vi "Pick A DOF.vi"(6 "LBCB Number":T1, 7 "Force Control Parameters":T3, 8 "error in (no error)":errorcluster, 9 "Force Group Priorities":T4, 10 "Forces Error \nWindow":dbl[](array[numeric]), 11 "Mixed Mode Convergence Status In":T2) -> (0 "error out":errorcluster, 3 "Mixed Mode Convergence Status Out":T2)   [LabVIEW 2009]
uses:
  Data Access Objects/Metadata/Cartesian Point.ctl
  Data Access Objects/Mixed Mode/Force Control Parameters.ctl
  Mixed Mode Convergence Status.ctl
  Data Access Objects/Metadata/LBCB Number.ctl
  Data Access Objects/Metadata/DAO Actions.ctl
  Apps/Yes No Button.ctl
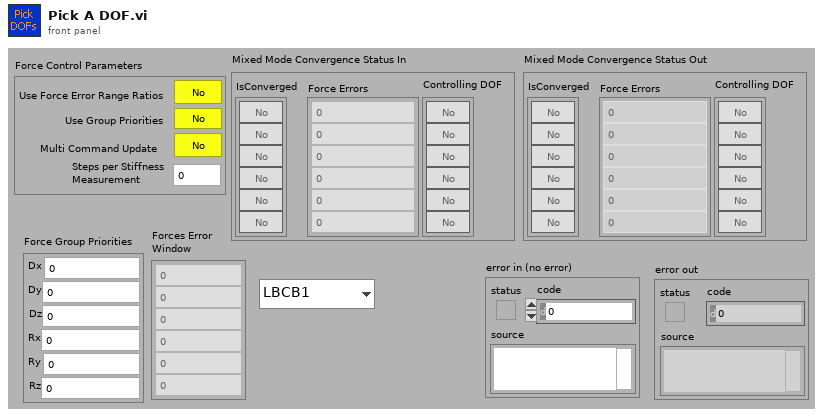
[diagram p1: front panel]
types:
  T1 = typedef "LBCB Number.ctl" = enum16{"LBCB1", "LBCB2"}
  T2 = typedef "Mixed Mode Convergence Status.ctl" = cluster{"IsConverged":bool[], "Force Errors":dbl[], "Controlling DOF":bool[]}
  T3 = typedef "Force Control Parameters.ctl" = cluster{"Use Force Error Range Ratios":bool, "Use Group Priorities":bool, "Multi Command Update":bool, "Steps per Stiffness \nMeasurement":i32}
  T4 = typedef "Cartesian Point.ctl" = cluster{"Dx":dbl, "Dy":dbl, "Dz":dbl, "Rx":dbl, "Ry":dbl, "Rz":dbl}
  T5 = typedef "Pick A DOF Strategy Types.ctl" = enum16{"Absolute Force Error", "Normalized Force Error", "Group Priorities Absolute", "Group Priorities Normalized", "Multi DOF Ramp Counting", "Multi DOF Ramp Counting Group", "Multi DOF Stiffness Test"}
  T6 = typedef "DAO Actions.ctl" = enum16{"Init", "Get", "Set"}
  T7 = typedef "Yes No Button.ctl" = bool
  T8 = typedef "Mixed Mode Multidof Status.ctl" = cluster{"Mixed Mode Multidof State":T9, "Multi DOF Ramp Count":i32, "Stiffness Tested":T7[][]}
  T9 = typedef "Mixed Mode Multidof State.ctl" = enum16{"Multidof", "Stiffness Test"}
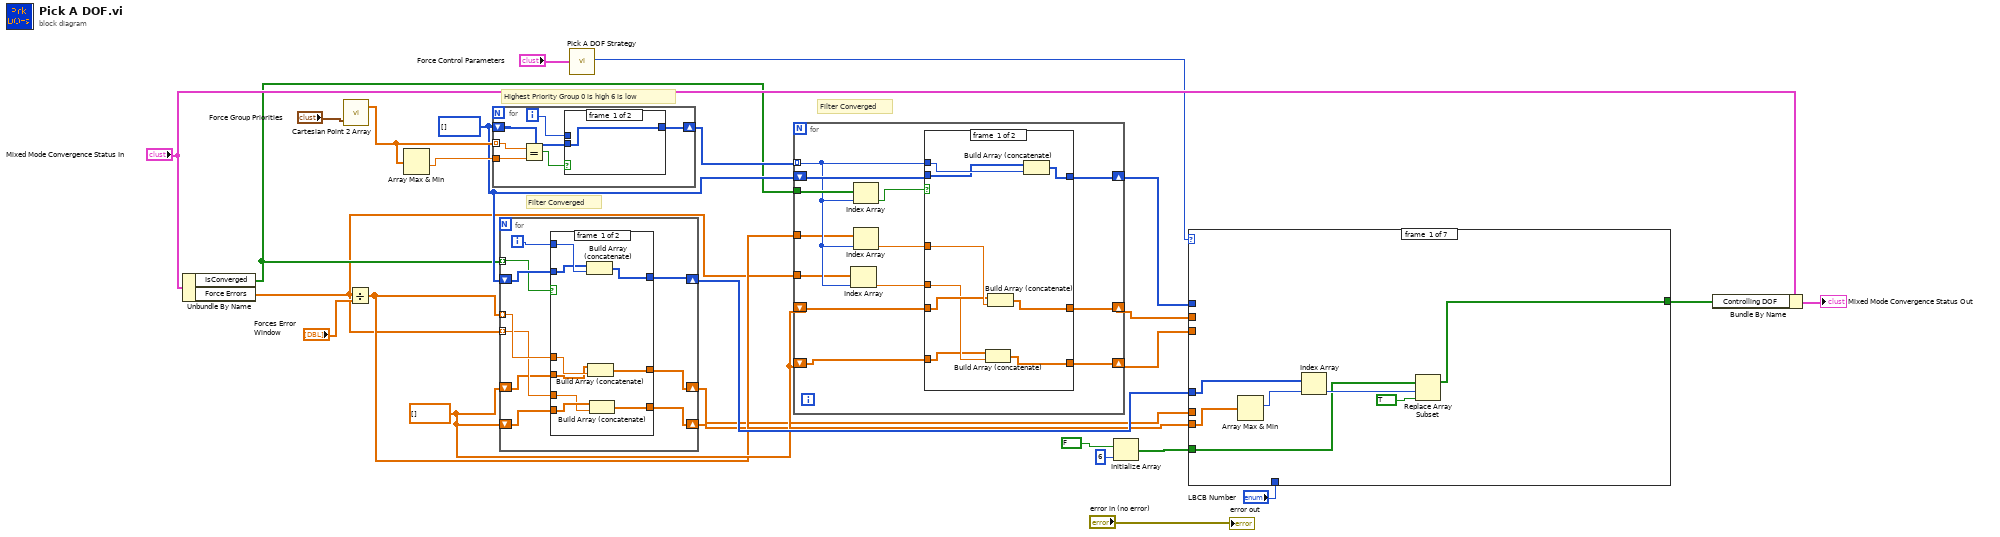
[diagram p0: block diagram]
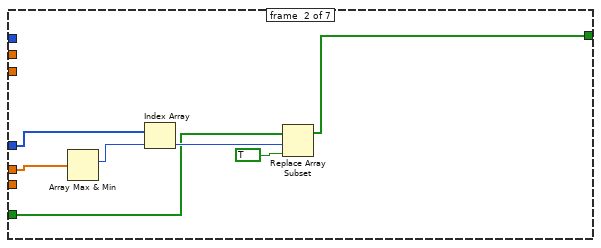
[diagram p2: hidden frame]
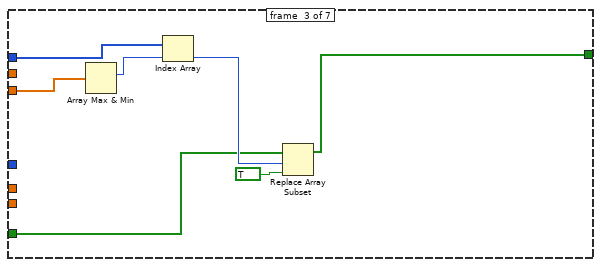
[diagram p3: hidden frame]
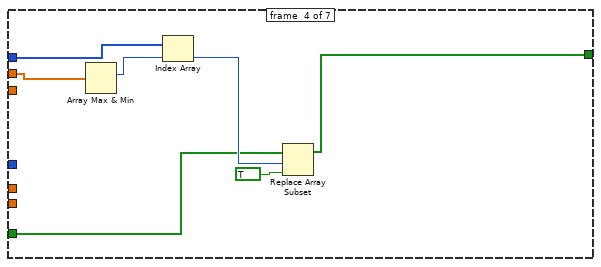
[diagram p4: hidden frame]
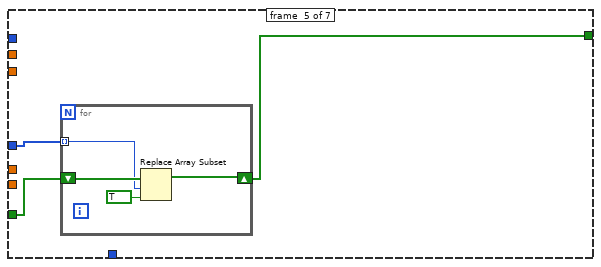
[diagram p5: hidden frame]
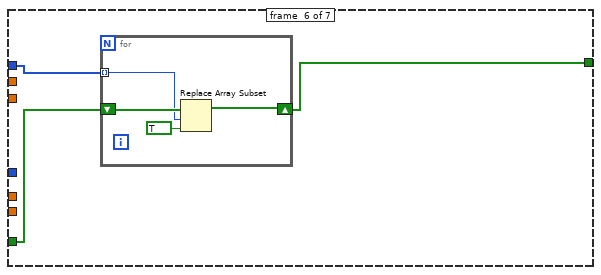
[diagram p6: hidden frame]
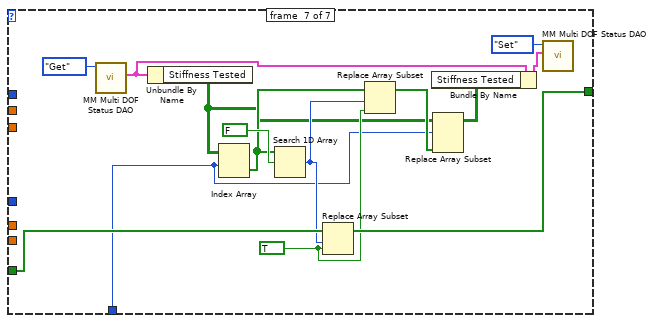
[diagram p7: hidden frame]
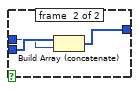
[diagram p10: hidden frame]
diagram:
  w10 = dbl[] []
  w17 = i32[] []
  # "Filter Converged"
  # "Filter Converged"
  # "Highest Priority Group 0 is high 6 is low"
  n1 = Unbundle By Name("Mixed Mode Convergence Status In") -> ("IsConverged"=w16:bool[], "Force Errors"=w1:dbl[])
  n2 = call "Cartesian Point 2 Array.vi"("Cart Disp"="Force Group Priorities") -> ("Array"=w20:dbl[])  [unwired: 2 in]
  n3 = Divide(x=w1, y="Forces Error \nWindow") -> (x/y=w9:dbl[])
  n4 = Array Max & Min(array=w20) -> (min value=w19:dbl)  [unwired: 3 out]
  n5 = for {
    shift-right: [w27] -> w18
    shift-left: w17 -> [w29]
    tunnel: w20 -> [w31] mode=indexing
    tunnel: w19 -> [w32]
    i -> [w28]
    n6 = Equal?(x=w31, y=w32) -> (x = y?=w30:bool)
    n7 = case shown="True" w30 {
      tunnel: w29 -> [w33 w35]
      tunnel: w28 -> [_ w34]
      tunnel: [w33 w36] -> w27
      frame #0 {
      }
      frame #1 {
        n8 = Build Array (concatenate)(w35, w34) -> (w36:i32[])
      }
    }
  }
  n9 = for {
    shift-right: [w44] -> w11
    shift-left: w17 -> [w45]
    tunnel: w16 -> [w43] mode=indexing
    shift-right: [w37] -> w5
    shift-left: w10 -> [w40]
    shift-right: [w38] -> w4
    shift-left: w10 -> [w39]
    tunnel: w9 -> [w42] mode=indexing
    tunnel: w1 -> [w41] mode=indexing
    i -> [w46]
    n10 = case shown="False" w43 {
      tunnel: w45 -> [w51 w58]
      tunnel: w46 -> [w52 _]
      tunnel: [w55 w58] -> w44
      tunnel: w42 -> [w50 _]
      tunnel: w41 -> [w47 _]
      tunnel: w40 -> [w49 w57]
      tunnel: w39 -> [w48 w56]
      tunnel: [w54 w56] -> w38
      tunnel: [w53 w57] -> w37
      frame #0 {
        n11 = Build Array (concatenate)(w51, w52) -> (w55:i32[])
        n12 = Build Array (concatenate)(w49, w50) -> (w53:dbl[])
        n13 = Build Array (concatenate)(w48, w47) -> (w54:dbl[])
      }
      frame #1 {
      }
    }
  }
  n14 = call "Pick A DOF Strategy.vi"("Force Control Parameters"="Force Control Parameters") -> ("Pick A DOF Strategy"=w14:T5)  [unwired: 10 in]
  n15 = for {
    tunnel: w16 -> [w69]
    tunnel: w18 -> [w67] mode=indexing
    shift-right: [w70] -> w12
    shift-left: w17 -> [w71]
    shift-right: [w59] -> w7
    shift-left: w10 -> [w62]
    shift-right: [w60] -> w6
    shift-left: w10 -> [w61]
    tunnel: w9 -> [w66]
    tunnel: w1 -> [w65]
    n16 = Index Array(array=w65, index=w67) -> (element=w63:dbl)
    n17 = Index Array(array=w69, index=w67) -> (element=w68:bool)
    n18 = Index Array(array=w66, index=w67) -> (element=w64:dbl)
    n19 = case shown="False" w68 {
      tunnel: w71 -> [w76 w83]
      tunnel: w67 -> [w77 _]
      tunnel: [w80 w83] -> w70
      tunnel: w64 -> [w75 _]
      tunnel: w63 -> [w73 _]
      tunnel: w62 -> [w74 w82]
      tunnel: w61 -> [w72 w81]
      tunnel: [w79 w81] -> w60
      tunnel: [w78 w82] -> w59
      frame #0 {
        n20 = Build Array (concatenate)(w72, w73) -> (w79:dbl[])
        n21 = Build Array (concatenate)(w74, w75) -> (w78:dbl[])
        n22 = Build Array (concatenate)(w76, w77) -> (w80:i32[])
      }
      frame #1 {
      }
    }
  }
  n23 = Initialize Array(FALSE, 6 ("dimension size")) -> (w13:bool[])
  n24 = case shown="\"Multi DOF Stiffness Test\"" w14 {
    tunnel: w13 -> [w86 w93 w101 w108 w113 w121 w137]
    tunnel: w12 -> [_ _ w99 w106 _ w119 _]
    tunnel: w11 -> [w87 w94 _ _ w114 _ _]
    tunnel: w7 -> [_ _ _ w105 _ _ _]
    tunnel: w6 -> [_ _ w98 _ _ _ _]
    tunnel: w5 -> [_ w91 _ _ _ _ _]
    tunnel: w4 -> [w85 _ _ _ _ _ _]
    tunnel: [w84 w92 w100 w107 w112 w120 w136] -> w3
    tunnel: "LBCB Number" -> [_ _ _ _ _ _ w130]
    frame #0 {
      n25 = Array Max & Min(array=w85) -> (max index (indices)=w90:i32)  [unwired: 3 out]
      n26 = Index Array(array=w87, index=w90) -> (element=w88:i32)
      n27 = Replace Array Subset(array=w86, new element=TRUE ("new element/subarray"), index=w88) -> (w84:bool[])
    }
    frame #1 {
      n28 = Array Max & Min(array=w91) -> (max index (indices)=w97:i32)  [unwired: 3 out]
      n29 = Index Array(array=w94, index=w97) -> (element=w95:i32)
      n30 = Replace Array Subset(array=w93, new element=TRUE ("new element/subarray"), index=w95) -> (w92:bool[])
    }
    frame #2 {
      n31 = Array Max & Min(array=w98) -> (max index (indices)=w104:i32)  [unwired: 3 out]
      n32 = Index Array(array=w99, index=w104) -> (element=w102:i32)
      n33 = Replace Array Subset(array=w101, new element=TRUE ("new element/subarray"), index=w102) -> (w100:bool[])
    }
    frame #3 {
      n34 = Array Max & Min(array=w105) -> (max index (indices)=w111:i32)  [unwired: 3 out]
      n35 = Index Array(array=w106, index=w111) -> (element=w109:i32)
      n36 = Replace Array Subset(array=w108, new element=TRUE ("new element/subarray"), index=w109) -> (w107:bool[])
    }
    frame #4 {
      n37 = for {
        tunnel: w114 -> [w117] mode=indexing
        shift-right: [w115] -> w112
        shift-left: w113 -> [w118]
        n38 = Replace Array Subset(array=w118, new element=TRUE ("new element/subarray"), index=w117) -> (w115:bool[])
      }
    }
    frame #5 {
      n39 = for {
        tunnel: w119 -> [w124] mode=indexing
        shift-right: [w122] -> w120
        shift-left: w121 -> [w125]
        n40 = Replace Array Subset(array=w125, new element=TRUE ("new element/subarray"), index=w124) -> (w122:bool[])
      }
    }
    frame #6 {
      w133 = TRUE ("new element/subarray")
      n41 = call "MM Multi DOF Status DAO.vi"("Actions"=DAO_Actions."Get") -> ("Mixed Mode Multidof Status Out"=w128:T8)  [unwired: 9 in, 1 out]
      n42 = Unbundle By Name(w128) -> ("Stiffness Tested"=w131:T7[][])
      n43 = Index Array(array=w131, index (row)=w130) -> (element=w135:T7[])  [unwired: 1 in]
      n44 = Search 1D Array(1D array=w135, element=T7 FALSE) -> (index of element=w134:i32)  [unwired: 1 in]
      n45 = Replace Array Subset(array=w137, new element=w133, index=w134) -> (w136:bool[])
      n46 = Replace Array Subset(array=w135, new element=w133, index=w134) -> (w132:T7[])
      n47 = Replace Array Subset(array=w131, new element=w132, index (row)=w130) -> (w126:T7[][])  [unwired: 1 in]
      n48 = Bundle By Name(cluster=w128, "Stiffness Tested"=w126) -> (w127:T8)
      n49 = call "MM Multi DOF Status DAO.vi"("Mixed Mode Multidof Status In"=w127, "Actions"=DAO_Actions."Set") -> ()  [unwired: 8 in, 2 out]
    }
  }
  n50 = Bundle By Name(cluster="Mixed Mode Convergence Status In", "Controlling DOF"=w3) -> (→"Mixed Mode Convergence Status Out":T2)
  "error out" <- "error in (no error)"
